vi "Prune.vi"(6 "File Extension":string="csv", 8 "Error In":errorcluster, 10 "Maximum File Count":i32, 11 "File In":refnum<file>) -> (0 "Error Out":errorcluster, 3 "File Out":refnum<file>)   [LabVIEW 2018, in "Toolkit.lvlib" / "File.lvlib"]
uses:
  File.lvlib
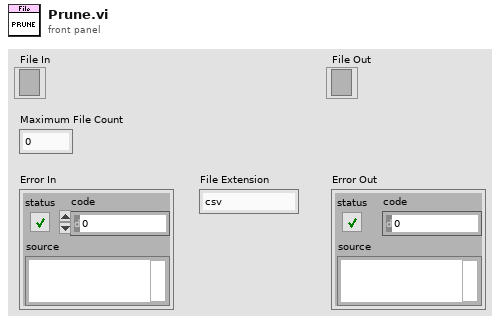
[diagram p1: front panel]
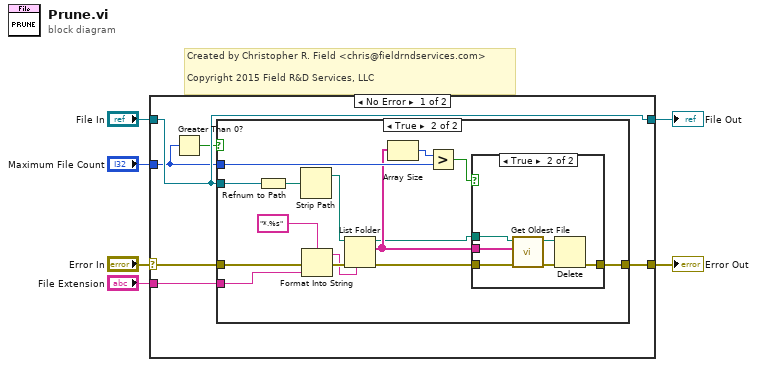
[diagram p0: block diagram]
diagram:
  # "Created by Christopher R. Field <chris@fieldrndservices.com>\n\nCopyright 2015 Field R&D Services, LLC"
  n1 = case shown="No Error" "Error In" {
    selector: "Error In" -> [w12 w37]
    tunnel: "File In" -> [w10 w36]
    tunnel: "Maximum File Count" -> [w9 _]
    tunnel: [w11 w37] -> w3
    tunnel: [w10 w36] -> w2
    tunnel: "File Extension" -> [w7 _]
    frame No Error {
      n2 = Greater Than 0?(x=w9) -> (x > 0?=w8:bool)
      n3 = case shown="True" w8 {
        tunnel: w12 -> [w13 w26]
        tunnel: w9 -> [_ w24]
        tunnel: [w13 w19] -> w11
        tunnel: w10 -> [_ w18]
        tunnel: w7 -> [_ w14]
        frame False {
        }
        frame True {
          n4 = Refnum to Path(1:w18) -> (0:w28:path)
          n5 = Strip Path(path=w28) -> (stripped path=w27:path)  [unwired: 1 out]
          n6 = Format Into String(format string="*.%s", error in=w26, w14) -> (resulting string=w15:string, error out=w17:errorcluster)  [unwired: 1 in]
          n7 = List Folder(path=w27, pattern=w15, error in=w17) -> (path out=w20:path, filenames=w21:string[], error out=w22:errorcluster)  [unwired: 1 in, 1 out]
          n8 = Array Size(array=w21) -> (size(s)=w25:i32)
          n9 = Greater?(x=w25, y=w24) -> (0:w23:bool)
          n10 = case shown="True" w23 {
            tunnel: w22 -> [w29 w35]
            tunnel: w21 -> [_ w33]
            tunnel: w20 -> [_ w34]
            tunnel: [w29 w30] -> w19
            frame False {
            }
            frame True {
              n11 = call "Get Oldest File.vi"("Error In"=w35, "File Names"=w33, "Folder"=w34) -> ("Error Out"=w31:errorcluster, "Oldest File"=w32:path)  [unwired: 7 in]
              n12 = Delete(path (use dialog)=w32, error in=w31) -> (error out=w30:errorcluster)  [unwired: 3 in, 2 out]
            }
          }
        }
      }
    }
    frame Error {
    }
  }
  "Error Out" <- w3
  "File Out" <- w2
